vi "Reset Actions.vi"(6 "State Loop Data in":T1, 11 "State in":refnum<class "State.lvclass">) -> (3 "State out":refnum<class "State.lvclass">, 4 "State Loop Data":T1)   [LabVIEW 2023, in "VolatusSeq.lvlib" / "State.lvclass"]
uses:
  State.lvclass
  State Loop Data.ctl
  Iteration Actions/Iteration Actions.lvclass
  Variables/Variables.lvclass
  Command.ctl
  Volatus/MessageQ/MessageQ.lvclass
  Format String/Format String.lvclass
  VolatusSeqConfig/Command Type.ctl
  messages/CmdDigital/Data.ctl
  messages/CmdAnalog/Data.ctl
  Send Type.ctl
  lv-vecto/Vecto/Channel DBL/Channel DBL.lvclass
  Transition/Transition.lvclass
  Sequence Time.ctl
  VolatusSeqConfig/Debug Flags.ctl
  VolatusSeq.lvlib
  VolatusSeqConfig/VolatusSeqConfig.lvlib
  messages/CmdDigital/CmdDigital.lvlib
  messages/CmdAnalog/CmdAnalog.lvlib
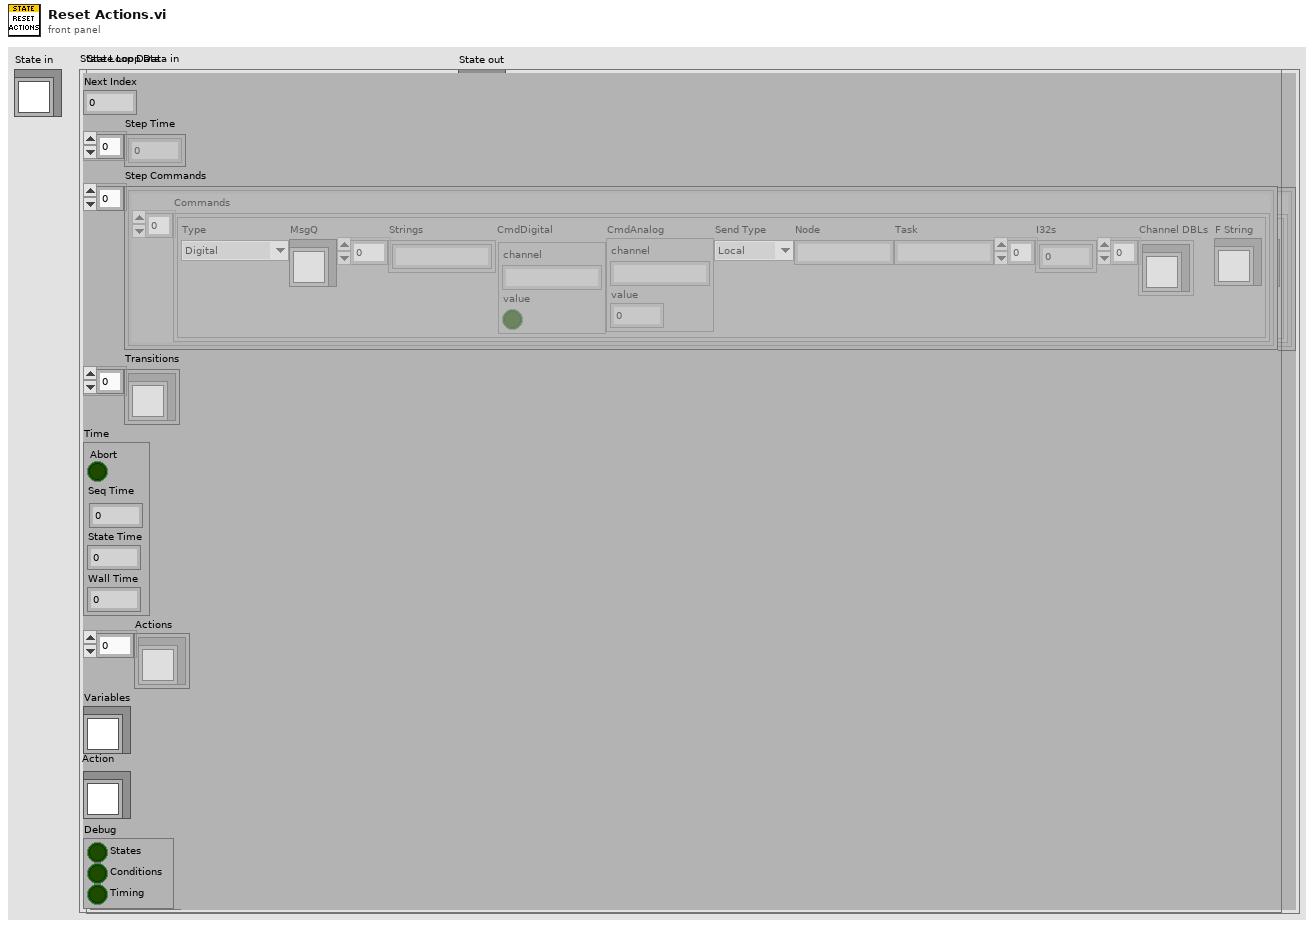
[diagram p1: front panel]
types:
  T1 = typedef "VolatusSeq.lvlib/State.lvclass/State Loop Data.ctl" = cluster{"Next Index":i32, "Step Time":dbl[], "Step Commands":cluster{"Commands":T2[]}[], "Transitions":refnum<class "Transition.lvclass">[], "Time":T7, "Actions":refnum<class "Iteration Actions.lvclass">[], "Variables":refnum<class "Variables.lvclass">, "Action":refnum<class "Iteration Actions.lvclass">, "Debug":T8}
  T2 = typedef "VolatusSeq.lvlib/Command.ctl" = cluster{"Type":T3, "MsgQ":refnum<class "MessageQ.lvclass">, "Strings":string[], "CmdDigital":T4, "CmdAnalog":T5, "Send Type":T6, "Node":string, "Task":string, "I32s":i32[], "Channel DBLs":refnum<class "Channel DBL.lvclass">[], "F String":refnum<class "Format String.lvclass">}
  T3 = typedef "VolatusSeqConfig.lvlib/Command Type.ctl" = enum16{"Digital", "Numeric", "Transition", "Stop", "StartLog", "StopLog", "Start", "Event", "Error", "HTTP", "ResetVar", "IncVar", "DecVar", "SaveVar", "LoadVar", "AddVar", "SubVar", "SetVar", "AddToVar"}
  T4 = typedef "CmdDigital.lvlib/Data.ctl" = cluster{"channel":string, "value":bool}
  T5 = typedef "CmdAnalog.lvlib/Data.ctl" = cluster{"channel":string, "value":dbl}
  T6 = typedef "VolatusSeq.lvlib/Send Type.ctl" = enum16{"Local", "Remote"}
  T7 = typedef "VolatusSeq.lvlib/Sequence Time.ctl" = cluster{"Abort":bool, "Seq Time":dbl, "State Time":dbl, "Wall Time":dbl}
  T8 = typedef "VolatusSeqConfig.lvlib/Debug Flags.ctl" = cluster{"States":bool, "Conditions":bool, "Timing":bool}
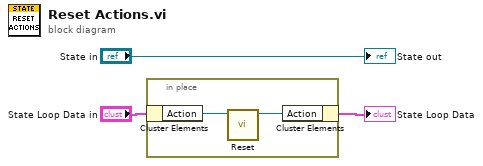
[diagram p0: block diagram]
diagram:
  n1 = in-place {
    n2 = in-place-cluster #1("State Loop Data in") -> ("Action"=w5:refnum<class "Iteration Actions.lvclass">)
    n3 = call "Reset.vi"("Iteration Actions in"=w5) -> ("Iteration Actions out"=w4:refnum<class "Iteration Actions.lvclass">)  [unwired: 9 in, 1 out]
    n4 = in-place-cluster #1("Action"=w4) -> (→"State Loop Data":T1)
  }
  "State out" <- "State in"
